vi "Read transactions.vi"(8 "error in (no error)":errorcluster, 11 "DbConnection in":refnum<class "ORM_DBC_dotNet.lvclass">) -> (0 "error out":errorcluster, 2 "transactions":refnum<k24>[](array[refnum]), 3 "DbConnection out":refnum<class "ORM_DBC_dotNet.lvclass">)   [LabVIEW 2020, in "ORM_DBC_dotNet.lvlib" / "ORM_DBC_dotNet.lvclass"]
uses:
  ORM_DBC_dotNet.lvclass
  System.Data
  ORM_DBC_dotNet.lvclass/ORM_DBC_dotNet.ctl
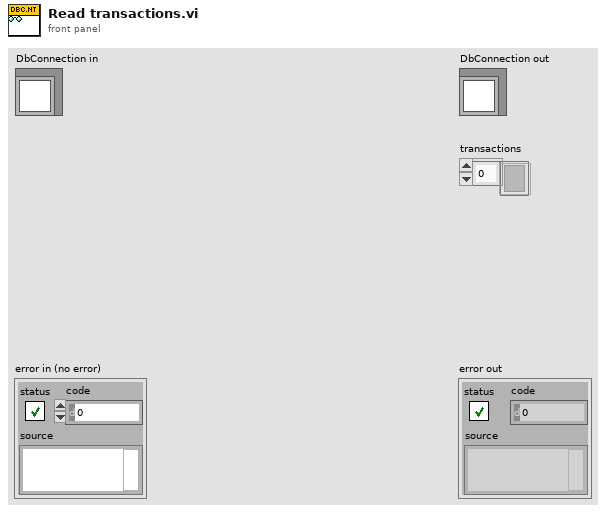
[diagram p1: front panel]
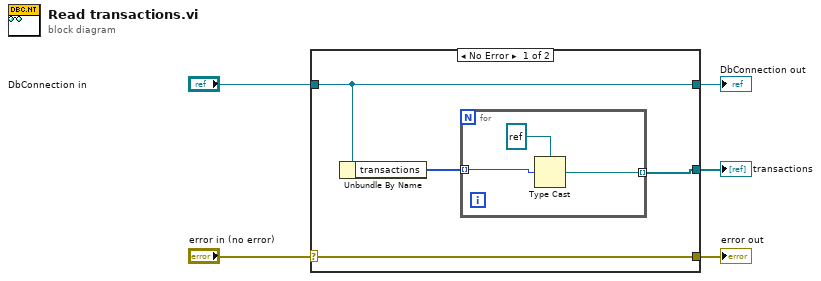
[diagram p0: block diagram]
diagram:
  n1 = case shown="No Error" "error in (no error)" {
    selector: "error in (no error)" -> [w9 w13]
    tunnel: [w9 w13] -> w4
    tunnel: [w8 w14] -> w2
    tunnel: "DbConnection in" -> [w8 w14]
    tunnel: [w6 _] -> w1
    frame No Error {
      n2 = Unbundle By Name(w8) -> ("transactions"=w7:u64[])
      n3 = for {
        tunnel: w7 -> [w12] mode=indexing
        tunnel: [w10] -> w6 mode=indexing
        n4 = Type Cast(type=refnum<k24> refnum ("BeginTransaction"), x=w12) -> (*(type *) &x=w10:refnum<k24>)
      }
    }
    frame Error {
    }
  }
  "error out" <- w4
  "DbConnection out" <- w2
  "transactions" <- w1
